vi "Enforce Robot Rules.vi"(5 "max V":dbl, 7 "Overrides":refnum<vi>, 8 "turn accel":dbl, 9 "Disable":bool, 10 "New Points":cluster{"x":dbl, "y":dbl, "th":dbl}[](array[cluster]), 11 "Original Points":cluster{"x":dbl, "y":dbl, "th":dbl}[](array[cluster])) -> (3 "Points out":cluster{"x":dbl, "y":dbl, "th":dbl}[](array[cluster]))   [LabVIEW 2019]
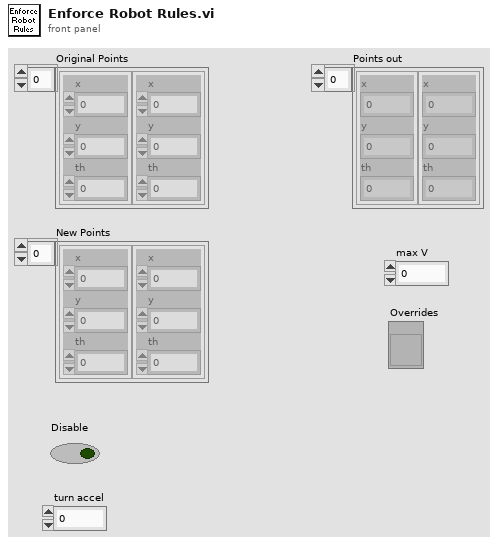
[diagram p1: front panel]
types:
  T1 = cluster{"Count":string, "Angular Multiplier":dbl, "1":bool, "Angular Multiplier 2":dbl}[]
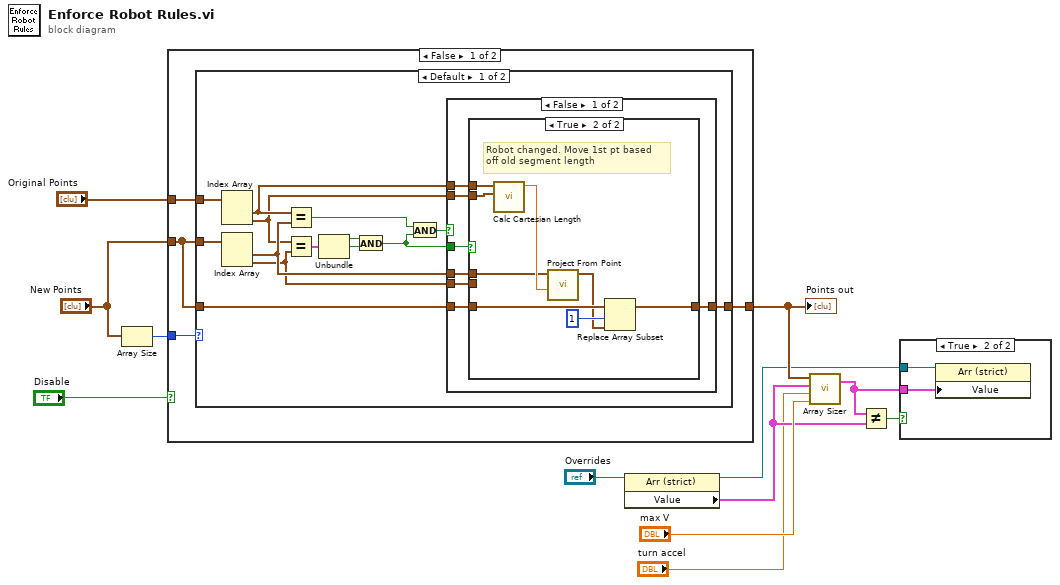
[diagram p0: block diagram]
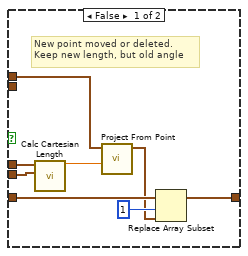
[diagram p3: hidden frame]
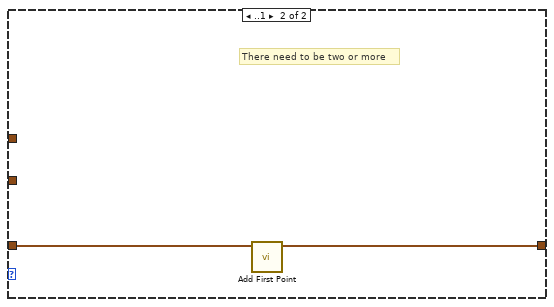
[diagram p5: hidden frame]
diagram:
  n1 = Array Size(array="New Points") -> (size(s)=w11:i32)
  n2 = case shown="False" "Disable" {
    tunnel: "Original Points" -> [w16 _]
    tunnel: w11 -> [w15 _]
    tunnel: [w14 w57] -> w8
    tunnel: "New Points" -> [w13 w57]
    frame False {
      n3 = case shown="Default" w15 {
        tunnel: w16 -> [w30 _]
        tunnel: w13 -> [w29 _]
        tunnel: [w27 w56] -> w14
        tunnel: w13 -> [w26 w55]
        frame Default {
          n4 = Index Array(array=w30) -> (element #1=w24:cluster{"x":dbl, "y":dbl, "th":dbl}, element #2=w21:cluster{"x":dbl, "y":dbl, "th":dbl})  [unwired: 2 in]
          n5 = Index Array(array=w29) -> (element #1=w23:cluster{"x":dbl, "y":dbl, "th":dbl}, element #2=w22:cluster{"x":dbl, "y":dbl, "th":dbl})  [unwired: 2 in]
          n6 = Equal?(x=w24, y=w23) -> (x = y?=w25:bool)
          n7 = Equal?(x=w21, y=w22) -> (x = y?=w20:cluster{"x":bool, "y":bool, "th":bool})
          n8 = Unbundle(w20) -> ("x"=w19:bool, "y"=w18:bool)  [unwired: 1 out]
          n9 = And(x=w19, y=w18) -> (x .and. y?=w17:bool)
          n10 = And(x=w25, y=w17) -> (x .and. y?=w28:bool)
          n11 = case shown="False" w28 {
            tunnel: [w33 w54] -> w27
            tunnel: w26 -> [w31 w54]
            tunnel: w17 -> [w35 _]
            tunnel: w24 -> [w37 _]
            tunnel: w21 -> [w36 _]
            tunnel: w23 -> [w34 _]
            tunnel: w22 -> [w32 _]
            frame False {
              n12 = case shown="True" w35 {
                tunnel: w37 -> [w40 w53]
                tunnel: w36 -> [_ w52]
                tunnel: w34 -> [w45 w47]
                tunnel: [w41 w50] -> w33
                tunnel: w32 -> [w44 _]
                tunnel: w31 -> [w42 w51]
                frame False {
                  # "New point moved or deleted.\nKeep new length, but old angle"
                  n13 = call "Calc Cartesian Length.vi"("Point 2"=w44, "Point 1"=w45) -> ("Length (f)"=w39:dbl)  [unwired: 8 in, 1 out]
                  n14 = call "Project From Point.vi"("distance"=w39, "Point In"=w40) -> ("Point Out"=w38:cluster{"x":dbl, "y":dbl, "th":dbl})  [unwired: 9 in]
                  n15 = Replace Array Subset(array=w42, new element=w38, index=1) -> (w41:cluster{"x":dbl, "y":dbl, "th":dbl}[])
                }
                frame True {
                  # "Robot changed. Move 1st pt based\noff old segment length"
                  n16 = call "Calc Cartesian Length.vi"("Point 2"=w52, "Point 1"=w53) -> ("Length (f)"=w48:dbl)  [unwired: 8 in, 1 out]
                  n17 = call "Project From Point.vi"("distance"=w48, "Point In"=w47) -> ("Point Out"=w46:cluster{"x":dbl, "y":dbl, "th":dbl})  [unwired: 9 in]
                  n18 = Replace Array Subset(array=w51, new element=w46, index=1) -> (w50:cluster{"x":dbl, "y":dbl, "th":dbl}[])
                }
              }
            }
            frame True {
              # "First two elements didn't\nchange. assume they are\ngood"
            }
          }
        }
        frame ..1 {
          # "There need to be two or more"
          n19 = call "Add First Point.vi"("Initial Points"=w55) -> ("Points"=w56:cluster{"x":dbl, "y":dbl, "th":dbl}[])  [unwired: 10 in]
        }
      }
    }
    frame True {
    }
  }
  "Points out" <- w8
  n20 = property class="Arr (strict)"(reference="Overrides") -> (reference out=w7:refnum<vi>, "Value"=w2:T1)  [unwired: 1 in, 1 out]
  n21 = call "Array Sizer.vi"("maxV"="max V", "turn accel"="turn accel", "Overrides"=w2, "Points out"=w8) -> ("Overrides 2"=w6:T1)  [unwired: 1 in]
  n22 = Not Equal?(x=w6, y=w2) -> (x != y?=w5:bool)
  n23 = case shown="True" w5 {
    tunnel: w6 -> [_ w59]
    tunnel: w7 -> [_ w58]
    frame False {
    }
    frame True {
      n24 = property class="Arr (strict)"(reference=w58, "Value"=w59) -> ()  [unwired: 1 in, 2 out]
    }
  }
